vi "LVDimInterface.dim_get_info.vi"(5 "error in (no error)":errorcluster) -> (11 "allowedNodes":string[](array[string]), 14 "versionNumber":i32, 15 "dimDnsNode":string, 16 "maxLocalDataSize":i32, 17 "pollingMode":bool, 18 "maxBufferSize":i32, 19 "error out":errorcluster)   [LabVIEW 2014, in "LVDimInterface.lvlib"]
doc: "Obtains information about DIM and some definitions used by CS-DIM servers.\n\nHistory: 16-DEC-2005, Dietrich Beck\n\nCopyright (C)\nGesellschaft für Schwerionenforschung, GSI\nPlanckstr. 1\n64291 Darmstadt\nGermany\n\nContact: D.Beck@gsi.de \n\nThis program is free software; you can redistribute it and/or modify it under the terms of the \nGNU General Public License as published by the Free Software Foundation; either version 2 of the license, or (at your option) any later version.\n\nThis program is distributed in the hope that it will be useful, but WITHOUT ANY WARRANTY; without even the implied warranty of MERCHANTABILITY or FITNESS FOR A PARTICULAR PURPOSE. See the GNU General License for more details (http://www.gnu.org).\n\nGesellschaft für Schwerionenforschung, GSI\nPlanckstr. 1, 64291 Darmstadt, Germany\nFor all questions and ideas contact D. Beck.\nLast update: 16-DEC-2005"
uses:
  LVDimInterface.lvlib
  bin/libDimWrapper.dll
  bin/libDimWrapper.so
  bin/libDimWrapperSPL.dll
panel:
  out "securityEnabled":bool
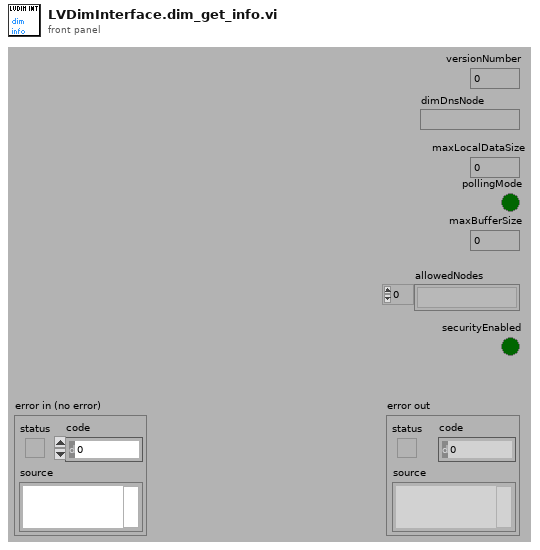
[diagram p1: front panel]
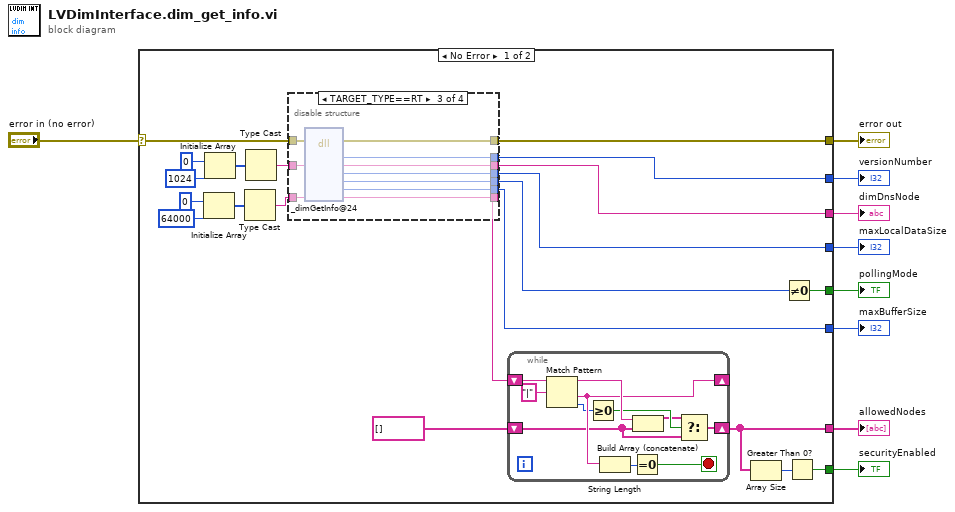
[diagram p0: block diagram]
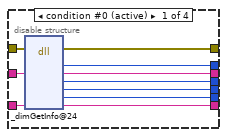
[diagram p2: hidden frame]
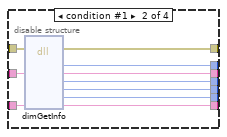
[diagram p3: hidden frame]
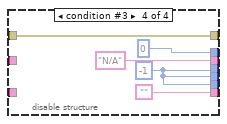
[diagram p4: hidden frame]
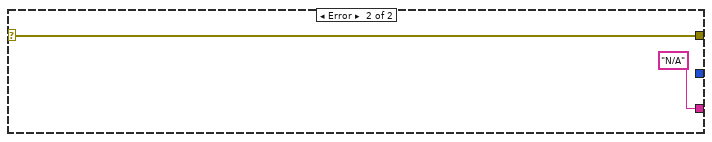
[diagram p5: hidden frame]
diagram:
  n1 = case shown="No Error" "error in (no error)" {
    selector: "error in (no error)" -> [w11 w77]
    tunnel: [w26 "N/A" ("dimDnsNode")] -> w9
    tunnel: [w25 _] -> w8
    tunnel: [w23 _] -> w7
    tunnel: [w22 _] -> w6
    tunnel: [w15 _] -> w5
    tunnel: [w13 _] -> w4
    tunnel: [w12 _] -> w3
    tunnel: [w10 w77] -> w1
    frame No Error {
      n2 = Initialize Array(u8 0, 64000 ("dimension size")) -> (w21:u8[])
      n3 = Initialize Array(u8 0, 1024 ("dimension size")) -> (w28:u8[])
      n4 = Type Cast(x=w21) -> (*(type *) &x=w18:string)  [unwired: 1 in]
      n5 = Type Cast(x=w28) -> (*(type *) &x=w27:string)  [unwired: 1 in]
      n6 = disable-structure "Conditional Disable Structure" shown="TARGET_TYPE==RT" {
        disable-tunnel: [w40 w50 w60 0 ("versionNumber")] -> w12
        disable-tunnel: w27 -> [w39 w49 w59 _]
        disable-tunnel: [w38 w48 w58 "N/A" ("dimDnsNode")] -> w26
        disable-tunnel: [w37 w47 w57 w63] -> w25
        disable-tunnel: [w36 w46 w56 w63] -> w24
        disable-tunnel: [w35 w45 w55 w63] -> w22
        disable-tunnel: w18 -> [w34 w44 w54 _]
        disable-tunnel: [w33 w43 w53 "" ("allowedNodes")] -> w16
        disable-tunnel: w11 -> [w32 w42 w52 w61]
        disable-tunnel: [w31 w41 w51 w61] -> w10
        frame condition #0 (active) {
          n7 = dll-call lib="D:/Git/CS-framework/CSlibraries-extern/DimLVEvent/bin/libDimWrapper.dll" fn="_dimGetInfo@24"(error in=w32, "dimDnsNode"=w39, "allowedNodes"=w34) -> (error out=w31:errorcluster, "versionNumber"=w40:i32, "dimDnsNode"=w38:string, "maxLocalDataSize"=w37:i32, "pollingMode"=w36:i32, "maxBufferSize"=w35:i32, "allowedNodes"=w33:string)  [unwired: 7 in, 1 out]
        }
        frame condition #1 {
          n8 = dll-call lib="D:/Git/CS-framework/CSlibraries/DimLVEvent/bin/libDimWrapper.so" fn="dimGetInfo"(error in=w42, "dimDnsNode"=w49, "allowedNodes"=w44) -> (error out=w41:errorcluster, "versionNumber"=w50:i32, "dimDnsNode"=w48:string, "maxLocalDataSize"=w47:i32, "pollingMode"=w46:i32, "maxBufferSize"=w45:i32, "allowedNodes"=w43:string)  [unwired: 7 in, 1 out]
        }
        frame condition #2 {
          n9 = dll-call lib="D:/Git/CS-framework/CSlibraries/DimLVEvent/bin/libDimWrapperSPL.dll" fn="_dimGetInfo@24" label="libDimWrapper.so:dimGetInfo"(error in=w52, "dimDnsNode"=w59, "allowedNodes"=w54) -> (error out=w51:errorcluster, "versionNumber"=w60:i32, "dimDnsNode"=w58:string, "maxLocalDataSize"=w57:i32, "pollingMode"=w56:i32, "maxBufferSize"=w55:i32, "allowedNodes"=w53:string)  [unwired: 7 in, 1 out]
        }
        frame condition #3 {
          w63 = -1 ("maxLocalDataSize")
        }
      }
      n10 = while {
        shift-right: [w72] -> _
        shift-left: w16 -> [w76]
        shift-right: [w71] -> w15
        shift-left: string[] [] -> [w66]
        stop <- w70 stop-if-true
        n11 = Match Pattern(string=w76, regular expression="|") -> (before substring=w73:string, after substring=w72:string, offset past match=w69:i32)  [unwired: 1 in, 1 out]
        n12 = Greater Or Equal To 0?(x=w69) -> (x >= 0?=w68:bool)
        n13 = String Length(string=w72) -> (length=w74:i32)
        n14 = Equal To 0?(x=w74) -> (x = 0?=w70:bool)
        n15 = Build Array (concatenate)(w73, w66) -> (w67:string[])
        n16 = Select(t=w67, s=w68, f=w66) -> (s? t:f=w71:string[])
      }
      n17 = Array Size(array=w15) -> (size(s)=w14:i32)
      n18 = Not Equal To 0?(x=w24) -> (x != 0?=w23:bool)
      n19 = Greater Than 0?(x=w14) -> (x > 0?=w13:bool)
    }
    frame Error {
    }
  }
  "error out" <- w1
  "versionNumber" <- w3
  "maxLocalDataSize" <- w8
  "dimDnsNode" <- w9
  "pollingMode" <- w7
  "maxBufferSize" <- w6
  "allowedNodes" <- w5
  "securityEnabled" <- w4
